vi "TrajectoryExecuteAbsolute.vi"(8 "Init":bool, 11 "End Pose ENG":T1={"TRANSLATION"={"X"=0.0, "Y"=0.0}, "ROTATION"={"VALUE"=0.0, "COS"=1.0, "SIN"=0.0}} {"ROTATION"."SIN" format="%13.4f"; "ROTATION"."COS" format="%13.4f"; "ROTATION"."VALUE" format="%13.4f"; "TRANSLATION"."Y" format="%14.3f"; "TRANSLATION"."X" format="%14.3f"}) -> (0 "AtReference":bool, 3 "Chassis Velocity Target":T4 {"vOmega" format="%10.3f"; "vY" format="%10.3f"; "vX" format="%10.3f"})   [LabVIEW 2023]
uses:
  <vilib>/Rock Robotics/WPI/ThirdParty/JAS_Junk/TrajLib/Trajectory_Library.lvlib
  TrajectoryGlobals.vi
  <vilib>/Rock Robotics/WPI/ThirdParty/JAS_Junk/TrajLib/TypeDef/CHASSIS_SPEEDS.ctl
  <vilib>/Rock Robotics/WPI/ThirdParty/JAS_Junk/TrajLib/TypeDef/TRANSLATION2D.ctl
  <vilib>/Rock Robotics/WPI/ThirdParty/JAS_Junk/TrajLib/TypeDef/ROTATION2D.ctl
  <vilib>/Rock Robotics/WPI/ThirdParty/JAS_Junk/TrajLib/TypeDef/POSE2D.ctl
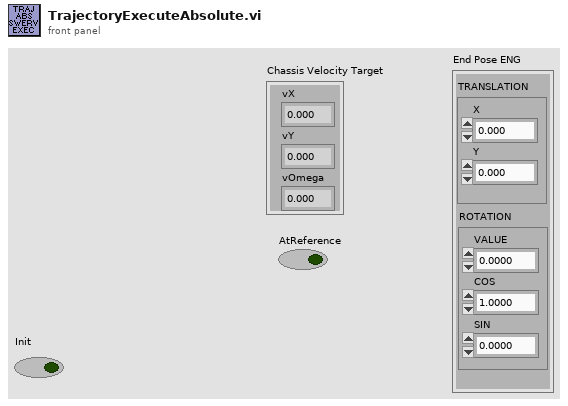
[diagram p1: front panel]
types:
  T1 = typedef "Trajectory_Library.lvlib/POSE2D.ctl" = cluster{"TRANSLATION":T2, "ROTATION":T3}
  T2 = typedef "Trajectory_Library.lvlib/TRANSLATION2D.ctl" = cluster{"X":dbl, "Y":dbl}
  T3 = typedef "Trajectory_Library.lvlib/ROTATION2D.ctl" = cluster{"VALUE":dbl, "COS":dbl, "SIN":dbl}
  T4 = typedef "Trajectory_Library.lvlib/CHASSIS_SPEEDS.ctl" = cluster{"vX":dbl, "vY":dbl, "vOmega":dbl}
  T5 = typedef "Trajectory_Library.lvlib/SWERVE_DRIVE_KINEMATICS.ctl" = cluster{"NumModules":i32, "InverseKinematics":T6, "ForwardKinematics":T6, "Modules":T2[], "PrevCoR":T2, "SavedModuleStates":T7[]}
  T6 = typedef "NI_Matrix.lvlib/RealMatrix.ctl" = dbl[][]
  T7 = typedef "Trajectory_Library.lvlib/SWERVE_DRIVE_MODULE_STATE.ctl" = cluster{"Speed":dbl, "Angle":T3}
  T8 = typedef "Trajectory_Library.lvlib/TRAJECTORY.ctl" = cluster{"TotalTImeSecs":dbl, "States":T9[]}
  T9 = typedef "Trajectory_Library.lvlib/TRAJ_STATE.ctl" = cluster{"TimeSeconds":dbl, "Velocity":dbl, "Acceleration":dbl, "POSE":T1, "Curvature":dbl}
  T10 = typedef "Trajectory_Library.lvlib/PID_TUNING.ctl" = cluster{"Kp":dbl, "Ki":dbl, "Kd":dbl, "MaximumIntegral":dbl, "MinimumIntegral":dbl, "IntegralZone":dbl}
  T11 = typedef "Trajectory_Library.lvlib/PROFILED_PID_CONTROLLER.ctl" = cluster{"Controller":T12, "Goal":T13, "Setpoint":T13, "Constraint":T14}
  T12 = typedef "Trajectory_Library.lvlib/PID_CONTROLLER.ctl" = cluster{"Kp":dbl, "Ki":dbl, "Kd":dbl, "Period":dbl, "Max_Integral":dbl, "Min_Integral":dbl, "Max_Input":dbl, "Min_Input":dbl, "Continuous":bool, "PositionError":dbl, "VelocityError":dbl, "PrevError":dbl, "Total_Integral":dbl, "PositionTolerance":dbl, "VelocityTolerance":dbl, "SetPoint":dbl, "Kf":dbl, "Prev_Deriv":dbl, "Prev_Deriv 2":dbl, "DerivativeFilter":bool, "Min_Output":dbl, "Max_Output":dbl, "Prev_F_P":dbl, "Prev_F_P_2":dbl, "AntiWindupActive":bool, "Measurement":dbl, "IntegralZone":dbl}
  T13 = typedef "Trajectory_Library.lvlib/TRAPEZOID_PROFILE_STATE.ctl" = cluster{"Position":dbl, "Velocity":dbl}
  T14 = typedef "Trajectory_Library.lvlib/TRAPEZOID_PROFILE_CONSTRAINT.ctl" = cluster{"MaxVelocity":dbl, "MaxAcceleration":dbl}
  T15 = typedef "Trajectory_Library.lvlib/HOLONOMIC_PACK_TUNING.ctl" = cluster{"X PID Tuning":T10, "Y PID Tuning":T10, "thetaProfiledPID_CTRL":T11}
  T16 = typedef "Trajectory_Library.lvlib/HOLONOMIC_DRV_CTRL.ctl" = cluster{"poseTolerance":T1, "poseError":T1, "Enabled":bool, "PID_xCtrl":T12, "PID_yCtrl":T12, "PROF_PID_thetaCtrl":T11, "RotationError":T3, "FirstRun":bool}
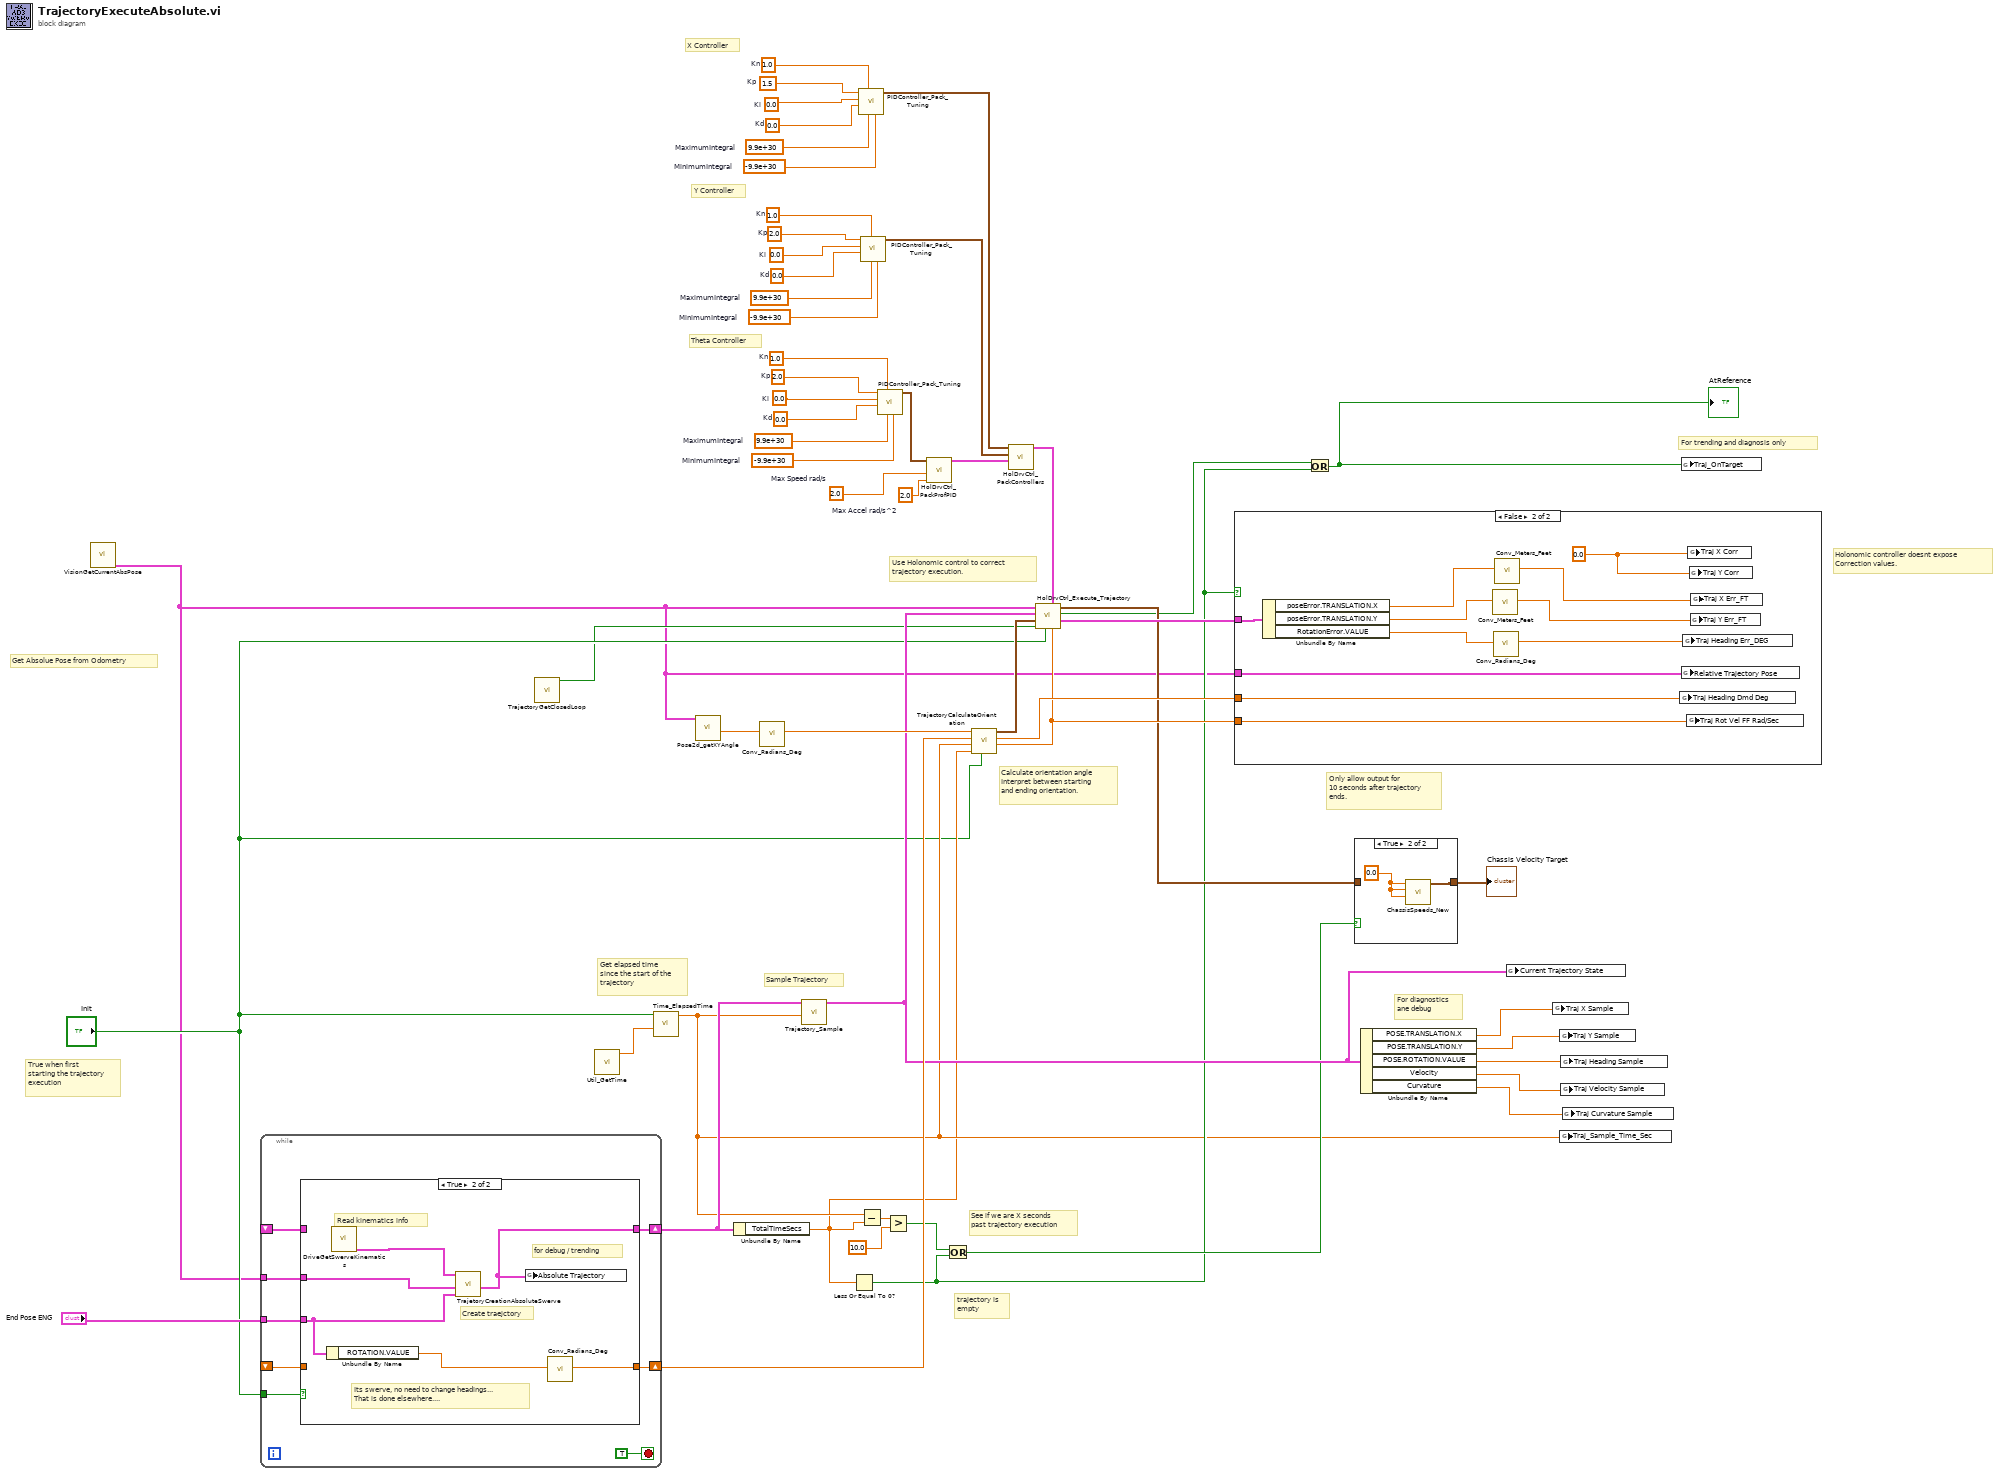
[diagram p0: block diagram]
diagram:
  w1 = 2.0  # Max Accel rad/s^2
  w2 = 2.0  # Max Speed rad/s
  w26 = 1.0  # Kn
  w29 = 2.0  # Kp
  w38 = 0.0  # Ki
  w39 = 0.0  # Kd
  w40 = 9.9e+30  # MaximumIntegral
  w41 = -9.9e+30  # MinimumIntegral
  w24 = 1.0  # Kn
  w27 = 1.5  # Kp
  w30 = 0.0  # Ki
  w31 = 0.0  # Kd
  w32 = 9.9e+30  # MaximumIntegral
  w33 = -9.9e+30  # MinimumIntegral
  w25 = 1.0  # Kn
  w28 = 2.0  # Kp
  w34 = 0.0  # Ki
  w35 = 0.0  # Kd
  w36 = 9.9e+30  # MaximumIntegral
  w37 = -9.9e+30  # MinimumIntegral
  # "trajectory is \nempty"
  # "Theta Controller"
  # "Y Controller"
  # "X Controller"
  # "Calculate orientation angle\nInterpret between starting\nand ending orientation."
  # "True when first\nstarting the trajectory\nexecution"
  # "Get elapsed time\nsince the start of the\ntrajectory"
  # "Holonomic controller doesnt expose\nCorrection values."
  # "Use Holonomic control to correct\ntrajectory execution."
  # "For trending and diagnosis only"
  # "For diagnostics\nane debug"
  # "Get Absolue Pose from Odometry"
  # "Sample Trajectory"
  # "See if we are X seconds \npast trajectory execution"
  # "Only allow output for\n10 seconds after trajectory\nends."
  n1 = call "VisionGetCurrentAbsPose.vi"() -> ("Current ABS Pose"=w3:T1)  [unwired: 9 in]
  n2 = while {
    tunnel: "Init" -> [w62]
    tunnel: w3 -> [w61]
    shift-right: [w60] -> w19
    shift-left: _ -> [w59]
    shift-right: [w58] -> w16
    shift-left: _ -> [w57]
    tunnel: "End Pose ENG" -> [w56]
    stop <- TRUE stop-if-true
    n3 = case shown="True" w62 {
      tunnel: w61 -> [_ w67]
      tunnel: [w65 w68] -> w60
      tunnel: w59 -> [w65 _]
      tunnel: [w64 w70] -> w58
      tunnel: w57 -> [w64 _]
      tunnel: w56 -> [_ w71]
      frame False {
      }
      frame True {
        # "for debug / trending"
        # "Read kinematics info"
        # "Its swerve, no need to change headings...\nThat is done elsewhere...."
        # "Create traejctory"
        n4 = Unbundle By Name(w71) -> ("ROTATION.VALUE"=w69:dbl)
        n5 = call "DriveGetSwerveKinematics.vi"() -> ("SWERVE_DRIVE_KINEMATICS"=w66:T5)  [unwired: 11 in]
        n6 = call "TrajetoryCreationAbsoluteSwerve.vi"("End Pose  ENG"=w71, "Current Pose SI"=w67, "SWERVE_DRIVE_KINEMATICS"=w66) -> ("Absolute Trajectory"=w68:T8)  [unwired: 6 in, 2 out]
        n7 = global write "TrajectoryGlobals.vi" "Absolute Trajectory"(w68) -> ()
        n8 = call <vilib>:"Conv_Radians_Deg.vi"("Radians"=w69) -> ("Degrees"=w70:dbl)  [unwired: 10 in]
      }
    }
  }
  n9 = call "TrajectoryGetClosedLoop.vi"() -> ("AUTO_CLOSED_LOOP"=w4:bool)  [unwired: 11 in]
  n10 = call <vilib>:"Util_GetTime.vi"() -> ("FPGA_Time_Seconds"=w52:dbl)  [unwired: 9 in, 2 out]
  n11 = call <vilib>:"Time_ElapsedTime.vi"("PassthroughTime_SEC"=w52, "Reset"="Init") -> ("Elapsed Time Sec"=w7:dbl)  [unwired: 9 in]
  n12 = call <vilib>:"Pose2d_getXYAngle.vi"("in POSE"=w3) -> ("Angle"=w18:dbl)  [unwired: 8 in, 2 out]
  n13 = Unbundle By Name(w19) -> ("TotalTImeSecs"=w6:dbl)
  n14 = call <vilib>:"Conv_Radians_Deg.vi"("Radians"=w18) -> ("Degrees"=w17:dbl)  [unwired: 10 in]
  n15 = call <vilib>:"Trajectory_Sample.vi"("Time"=w7, "InputTRAJECTORY"=w19) -> ("OutputTRAJ_STATE"=w15:T9)  [unwired: 9 in]
  n16 = Less Or Equal To 0?(x=w6) -> (x <= 0?=w8:bool)
  n17 = call <vilib>:"PIDController_Pack_Tuning.vi"("MinimumIntegral"=w33, "MaximumIntegral"=w32, "Kn"=w24, "Kd"=w31, "Ki"=w30, "Kp"=w27) -> ("PID Tuning"=w42:T10)  [unwired: 5 in]
  n18 = Subtract(x=w7, y=w6) -> (x-y=w55:dbl)
  n19 = call <vilib>:"PIDController_Pack_Tuning.vi"("MinimumIntegral"=w37, "MaximumIntegral"=w36, "Kn"=w25, "Kd"=w35, "Ki"=w34, "Kp"=w28) -> ("PID Tuning"=w43:T10)  [unwired: 5 in]
  n20 = call <vilib>:"PIDController_Pack_Tuning.vi"("MinimumIntegral"=w41, "MaximumIntegral"=w40, "Kn"=w26, "Kd"=w39, "Ki"=w38, "Kp"=w29) -> ("PID Tuning"=w23:T10)  [unwired: 5 in]
  n21 = Greater?(x=w55, y=10.0) -> (0:w12:bool)
  n22 = call <vilib>:"HolDrvCtrl_PackProfPID.vi"("Max Accel"=w1, "Max Speed"=w2, "Theta PID Tuning"=w23) -> ("Theta PID CONTROLLER"=w44:T11)  [unwired: 8 in]
  n23 = Or(x=w12, y=w8) -> (x .or. y?=w11:bool)
  n24 = call "TrajectoryCalculateOrientation.vi"("Init"="Init", "Total Trajectory Time Sec"=w6, "Elapsed Traj Time Sec"=w7, "End Orientation Demand DEG"=w16, "Starting Orientation  DEG"=w17) -> ("Rotational Velocity Rad Per Sec"=w20:dbl, "Orientation Demand Deg"=w46:dbl, "Orientation Demand"=w22:T3)  [unwired: 4 in]
  n25 = call <vilib>:"HolDrvCtrl_PackControllers.vi"("thetaProfiledPID_CTRL"=w44, "Y PID Tuning"=w43, "X PID Tuning"=w42) -> ("HOLONOMIC_CTRL_PACK_TUNING"=w45:T15)  [unwired: 8 in]
  n26 = call <vilib>:"HolDrvCtrl_Execute_Trajectory.vi"("Rotational Velocity Feedforward \nRad/Sec"=w20, "HOLONOMIC_CTRL_PACK_TUNING"=w45, "Reset"="Init", "Enable"=w4, "angleRef"=w22, "desiredTrajState"=w15, "currentPose"=w3) -> ("outHOLONOMIC_DRV_CTRL"=w21:T16, "AtReference"=w10:bool, "calcChassisSpeed"=w13:T4)  [unwired: 2 in]
  n27 = case shown="False" w8 {
    tunnel: w46 -> [_ w81]
    tunnel: w21 -> [_ w75]
    tunnel: w20 -> [_ w74]
    tunnel: w3 -> [_ w72]
    frame True {
    }
    frame False {
      w82 = 0.0 ("Y Corr")
      n28 = Unbundle By Name(w75) -> ("poseError.TRANSLATION.X"=w79:dbl, "poseError.TRANSLATION.Y"=w78:dbl, "RotationError.VALUE"=w73:dbl)
      n29 = call <vilib>:"Conv_Meters_Feet.vi"("Meters"=w78) -> ("Feet"=w77:dbl)  [unwired: 10 in]
      n30 = call <vilib>:"Conv_Radians_Deg.vi"("Radians"=w73) -> ("Degrees"=w80:dbl)  [unwired: 10 in]
      n31 = call <vilib>:"Conv_Meters_Feet.vi"("Meters"=w79) -> ("Feet"=w76:dbl)  [unwired: 10 in]
      n32 = global write "TrajectoryGlobals.vi" "Traj Heading Dmd Deg"(w81) -> ()
      n33 = global write "TrajectoryGlobals.vi" "Relative Trajectory Pose"(w72) -> ()
      n34 = global write "TrajectoryGlobals.vi" "Traj Heading Err_DEG"(w80) -> ()
      n35 = global write "TrajectoryGlobals.vi" "Traj Rot Vel FF Rad/Sec"(w74) -> ()
      n36 = global write "TrajectoryGlobals.vi" "Traj X Corr"(w82) -> ()
      n37 = global write "TrajectoryGlobals.vi" "Traj Y Corr"(w82) -> ()
      n38 = global write "TrajectoryGlobals.vi" "Traj Y Err_FT"(w77) -> ()
      n39 = global write "TrajectoryGlobals.vi" "Traj X Err_FT"(w76) -> ()
    }
  }
  n40 = Or(x=w10, y=w8) -> (x .or. y?=w9:bool)
  "AtReference" <- w9
  n41 = case shown="True" w11 {
    tunnel: w13 -> [w83 _]
    tunnel: [w83 w84] -> w53
    frame False {
    }
    frame True {
      w85 = 0.0 ("vX")
      n42 = call <vilib>:"ChassisSpeeds_New.vi"("vAngular"=w85, "vY"=w85, "vX"=w85) -> ("CHASSIS"=w84:T4)  [unwired: 8 in]
    }
  }
  "Chassis Velocity Target" <- w53
  n43 = Unbundle By Name(w15) -> ("POSE.TRANSLATION.X"=w51:dbl, "POSE.TRANSLATION.Y"=w50:dbl, "POSE.ROTATION.VALUE"=w49:dbl, "Velocity"=w48:dbl, "Curvature"=w47:dbl)
  n44 = global write "TrajectoryGlobals.vi" "Current Trajectory State"(w15) -> ()
  n45 = global write "TrajectoryGlobals.vi" "Traj X Sample"(w51) -> ()
  n46 = global write "TrajectoryGlobals.vi" "Traj Y Sample"(w50) -> ()
  n47 = global write "TrajectoryGlobals.vi" "Traj_Sample_Time_Sec"(w7) -> ()
  n48 = global write "TrajectoryGlobals.vi" "Traj Heading Sample"(w49) -> ()
  n49 = global write "TrajectoryGlobals.vi" "Traj Velocity Sample"(w48) -> ()
  n50 = global write "TrajectoryGlobals.vi" "Traj Curvature Sample"(w47) -> ()
  n51 = global write "TrajectoryGlobals.vi" "Traj_OnTarget"(w9) -> ()
